vi "Write Log Line.vi"(10 "log line":string, 11 "direct handler in":refnum<class "Direct Handler.lvclass">) -> (0 "error out":errorcluster, 3 "direct handler out":refnum<class "Direct Handler.lvclass">)   [LabVIEW 2024, in "Logging.lvlib" / "Direct Handler.lvclass"]
uses:
  Direct Handler.lvclass
  <vilib>/ErrorRing/Error Ring.xnode
  Utilities/Utilities.lvlib
panel:
  # "Connector Pane"
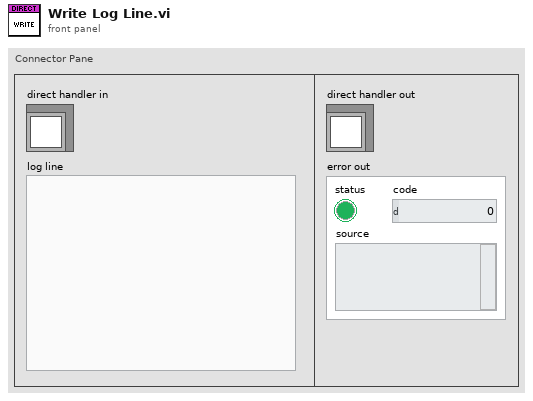
[diagram p1: front panel]
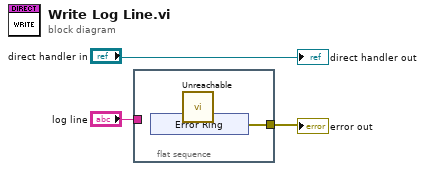
[diagram p0: block diagram]
diagram:
  n1 = flat-sequence {
    tunnel: "log line" -> [_]
    tunnel: [w4] -> w3
    frame #0 {
      n2 = xnode "Error Ring"() -> ("error out"=w4:errorcluster)
      n3 = call "Unreachable.vi"() -> ()  [unwired: 12 in]
    }
  }
  "direct handler out" <- "direct handler in"
  "error out" <- w3
